vi "Read and write vision info.vi"() -> ()   [LabVIEW 2013]
panel:
  out "Bitdepth":string
  out "ROI 2":T1={"Width"={"Value"=618.0, "Min"=1.0, "Max"=3000.0, "StepSize"=1.0, "Tolerance"=0.0, "valueactual"=0.0}, "Height"={"Value"=813.0, "Min"=1.0, "Max"=3000.0, "StepSize"=1.0, "Tolerance"=0.0, "valueactual"=0.0}, "OffsetX"={"Value"=0.0, "Min"=0.0, "Max"=1000.0, "StepSize"=1.0, "Tolerance"=0.0, "valueactual"=0.0}, "OffsetY"={"Value"=0.0, "Min"=0.0, "Max"=1000.0, "StepSize"=1.0, "Tolerance"=0.0, "valueactual"=0.0}}
  out "Keys":string[](array[string])
  in  "Image path":path
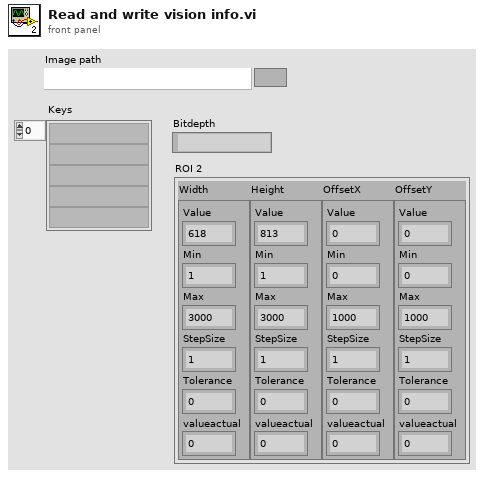
[diagram p1: front panel]
types:
  T1 = cluster{"Width":cluster{"Value":dbl, "Min":dbl, "Max":dbl, "StepSize":dbl, "Tolerance":dbl, "valueactual":dbl}, "Height":cluster{"Value":dbl, "Min":dbl, "Max":dbl, "StepSize":dbl, "Tolerance":dbl, "valueactual":dbl}, "OffsetX":cluster{"Value":dbl, "Min":dbl, "Max":dbl, "StepSize":dbl, "Tolerance":dbl, "valueactual":dbl}, "OffsetY":cluster{"Value":dbl, "Min":dbl, "Max":dbl, "StepSize":dbl, "Tolerance":dbl, "valueactual":dbl}}
  T2 = typedef "IMAQ Image.ctl" = refnum<image>
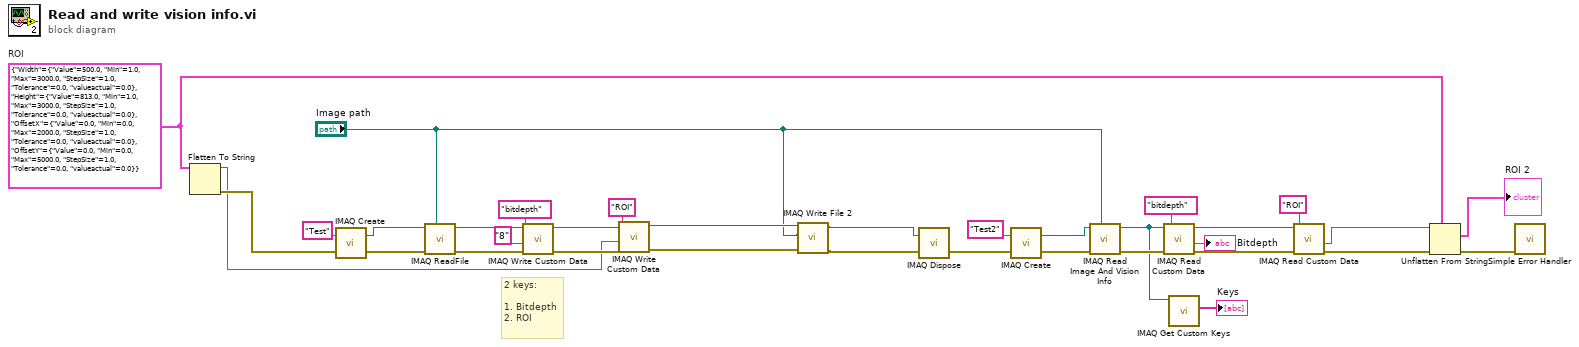
[diagram p0: block diagram]
diagram:
  w17 = T1 {"Width"={"Value"=500.0, "Min"=1.0, "Max"=3000.0, "StepSize"=1.0, "Tolerance"=0.0, "valueactual"=0.0}, "Height"={"Value"=813.0, "Min"=1.0, "Max"=3000.0, "StepSize"=1.0, "Tolerance"=0.0, "valueactual"=0.0}, "OffsetX"={"Value"=0.0, "Min"=0.0, "Max"=2000.0, "StepSize"=1.0, "Tolerance"=0.0, "valueactual"=0.0}, "OffsetY"={"Value"=0.0, "Min"=0.0, "Max"=5000.0, "StepSize"=1.0, "Tolerance"=0.0, "valueactual"=0.0}}  # ROI
  # "2 keys:\n\n1. Bitdepth\n2. ROI"
  n1 = Flatten To String(anything=w17) -> (data string=w11:string, error out=w30:errorcluster)  [unwired: 3 in, 1 out]
  n2 = call "IMAQ Create"("Image Name"="Test", "error in (no error)"=w30) -> ("New Image"=w34:T2, "error out"=w33:errorcluster)  [unwired: 3 in]
  n3 = call "IMAQ ReadFile"("File Path"="Image path", "error in (no error)"=w33, "Image"=w34) -> ("error out"=w31:errorcluster, "Image Out"=w32:T2)  [unwired: 4 in, 3 out]
  n4 = call "IMAQ Write Custom Data"("error in (no error)"=w31, "Custom Data In"="8", "Key"="bitdepth", "Image"=w32) -> ("error out"=w14:errorcluster, "Image Out"=w13:T2)  [unwired: 6 in]
  n5 = call "IMAQ Write Custom Data"("error in (no error)"=w14, "Custom Data In"=w11, "Key"="ROI", "Image"=w13) -> ("error out"=w9:errorcluster, "Image Out"=w10:T2)  [unwired: 6 in]
  n6 = call-poly "IMAQ Write File 2"("error in (no error)"=w9, "File Path"="Image path", "Image"=w10) -> ("error out"=w21:errorcluster, "Image Out (duplicate)"=w22:T2)  [unwired: 7 in]
  n7 = call "IMAQ Dispose"("Image"=w22, "error in (no error)"=w21) -> ("error out"=w26:errorcluster)  [unwired: 4 in]
  n8 = call "IMAQ Create"("Image Name"="Test2", "error in (no error)"=w26) -> ("New Image"=w24:T2, "error out"=w27:errorcluster)  [unwired: 3 in]
  n9 = call "IMAQ Read Image And Vision Info"("File Path"="Image path", "error in (no error)"=w27, "Image"=w24) -> ("error out"=w25:errorcluster, "Image Out"=w19:T2)  [unwired: 6 in, 1 out]
  n10 = call "IMAQ Read Custom Data"("error in (no error)"=w25, "Key"="bitdepth", "Image"=w19) -> ("error out"=w7:errorcluster, "Custom Data Out"=→"Bitdepth":string, "Image (duplicate)"=w8:T2)  [unwired: 6 in]
  n11 = call "IMAQ Get Custom Keys"("Image"=w19) -> ("Keys"=→"Keys":string[])  [unwired: 7 in, 3 out]
  n12 = call "IMAQ Read Custom Data"("error in (no error)"=w7, "Key"="ROI", "Image"=w8) -> ("error out"=w5:errorcluster, "Custom Data Out"=w6:string)  [unwired: 6 in, 1 out]
  n13 = Unflatten From String(type=w17, binary string=w6, error in (no error)=w5) -> (value=→"ROI 2":T1, error out=w23:errorcluster)  [unwired: 2 in, 1 out]
  n14 = call <vilib>:"Simple Error Handler.vi"("error in (no error)"=w23) -> ()  [unwired: 4 in, 5 out]
